vi "S2C_Shared_Proc_ManageClose.vi"(7 "VI_Ref":refnum<vi>, 8 "Error In":errorcluster, 11 "Q-Ref":refnum<queue>) -> (0 "Error Out":errorcluster, 3 "Exit?":bool)   [LabVIEW 2024]
uses:
  S2C_Shared_Proc_Globals.vi
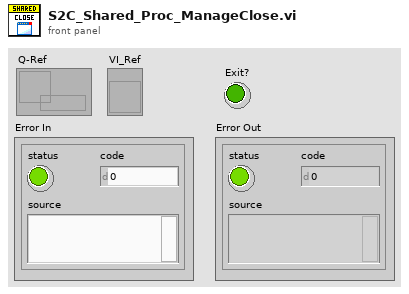
[diagram p1: front panel]
types:
  T1 = cluster{"Caller-Q":refnum<queue>, "Command":string, "Return":string, "Data":variant, "Timeout":dbl}
  T2 = enum32{"Invalid", "Standard", "Closed", "Hidden", "Minimized", "Maximized"}
  T3 = enum32{"Bad", "Idle", "Run top level", "Running"}
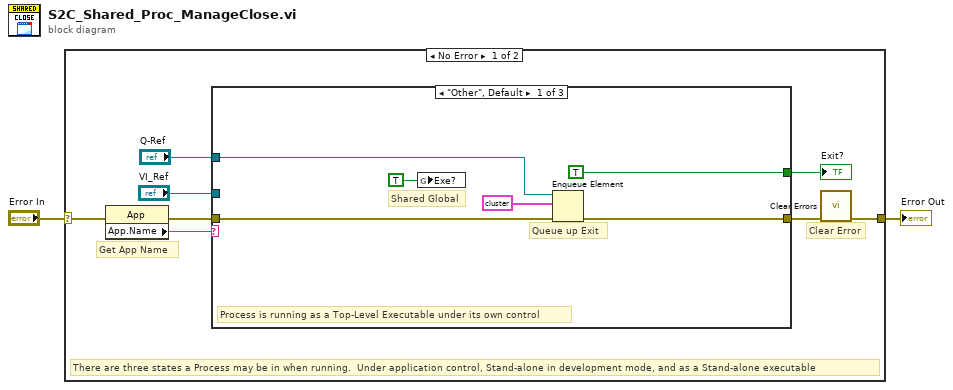
[diagram p0: block diagram]
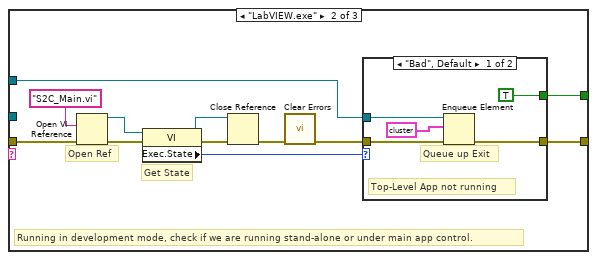
[diagram p2: hidden frame]
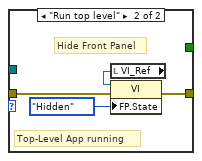
[diagram p3: hidden frame]
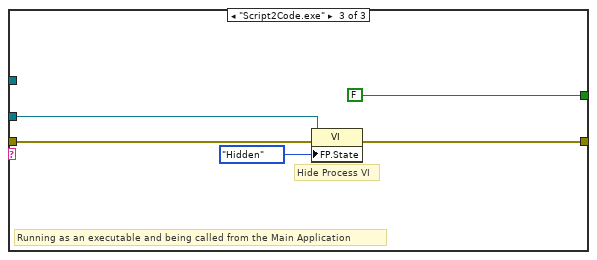
[diagram p4: hidden frame]
diagram:
  n1 = case shown="No Error" "Error In" {
    selector: "Error In" -> [w9 w43]
    tunnel: [w10 w43] -> w1
    frame No Error {
      # "Get App Name"
      # "Clear Error"
      # "There are three states a Process may be in when running.  Under application control, Stand-alone in development mode, and as a Stand-alone executable"
      n2 = property class="App"(error in=w9) -> (error out=w7:errorcluster, "App.Name"=w8:string)  [unwired: 1 in, 1 out]
      n3 = case shown="\"Other\", Default" w8 {
        tunnel: w7 -> [w15 w26 w41]
        tunnel: "VI_Ref" -> [_ _ w40]
        tunnel: [w11 w23 w39] -> w5
        tunnel: [TRUE w22 FALSE ("Exit?")] -> w4
        tunnel: "Q-Ref" -> [w14 w21 _]
        frame "Other", Default {
          # "Process is running as a Top-Level Executable under its own control"
          # "Shared Global"
          # "Queue up Exit"
          n4 = global write "S2C_Shared_Proc_Globals.vi" "Exe?"(TRUE ("Exe?")) -> ()
          n5 = Enqueue Element(queue=w14, element=T1 {"Caller-Q"=refnum, "Command"="^Exit", "Return"="", "Data"=variant, "Timeout"=0.0}, error in (no error)=w15) -> (error out=w11:errorcluster)  [unwired: 1 in, 2 out]
        }
        frame "LabVIEW.exe" {
          # "Running in development mode, check if we are running stand-alone or under main app control."
          # "Get State"
          # "Open Ref"
          n6 = Open VI Reference(vi path="S2C_Main.vi" ("element"), error in (no error)=w26) -> (vi reference=w27:refnum<vi>, error out=w28:errorcluster)  [unwired: 4 in]
          n7 = property class="VI"(reference=w27, error in=w28) -> (reference out=w19:refnum<vi>, error out=w20:errorcluster, "Exec.State"=w24:T3)
          n8 = Close Reference(reference=w19, error in (no error)=w20) -> (error out=w18:errorcluster)
          n9 = call <vilib>:"Clear Errors.vi"("error in (no error)"=w18) -> ("error out"=w17:errorcluster)  [unwired: 5 in, 1 out]
          n10 = case shown="\"Bad\", Default" w24 {
            tunnel: [w32 w37] -> w23
            tunnel: [TRUE _] -> w22
            tunnel: w17 -> [w33 w35]
            tunnel: w21 -> [w31 _]
            frame "Bad", Default {
              # "Top-Level App not running"
              # "Queue up Exit"
              n11 = Enqueue Element(queue=w31, element=T1 {"Caller-Q"=refnum, "Command"="^Exit", "Return"="", "Data"=variant, "Timeout"=0.0}, error in (no error)=w33) -> (error out=w32:errorcluster)  [unwired: 1 in, 2 out]
            }
            frame "Run top level" {
              # "Hide Front Panel"
              # "Top-Level App running"
              n12 = local read "VI_Ref"() -> (w34:refnum<vi>)
              n13 = property class="VI"(reference=w34, error in=w35, "FP.State"=T2."Hidden" ("Front Panel Window:State")) -> (error out=w37:errorcluster)  [unwired: 1 out]
            }
          }
        }
        frame "Script2Code.exe" {
          # "Running as an executable and being called from the Main Application"
          # "Hide Process VI"
          n14 = property class="VI"(reference=w40, error in=w41, "FP.State"=T2."Hidden" ("Front Panel Window:State")) -> (error out=w39:errorcluster)  [unwired: 1 out]
        }
      }
      "Exit?" <- w4
      n15 = call <vilib>:"Clear Errors.vi"("error in (no error)"=w5) -> ("error out"=w10:errorcluster)  [unwired: 5 in, 1 out]
    }
    frame Error {
    }
  }
  "Error Out" <- w1
